vi "Read.vi"(6 "Append Index":i32, 8 "error in (no error)":errorcluster, 11 "DAT in":refnum<class "Data.DAT.lvclass">) -> (0 "error out":errorcluster, 1 "Notes":string, 2 "Data (Dictionary)":T1[](array[typedef]), 3 "DAT out":refnum<class "Data.DAT.lvclass">, 5 "Path out":path)   [LabVIEW 2020, in "Data.DAT.lvclass"]
uses:
  Data.DAT.lvclass
  Data/Data.lvclass
  <vilib>/Utility/file.llb/Read Delimited Spreadsheet (string).vi
  C:/Users/Maya/Documents/GitHub/LV-to-ITX/src/Data/Data.lvclass
  C:/Users/Maya/Documents/GitHub/LV-to-ITX/src/Data.DAT/Data.DAT.lvclass
  Data/Typedefs/Dictionary--cluster.ctl
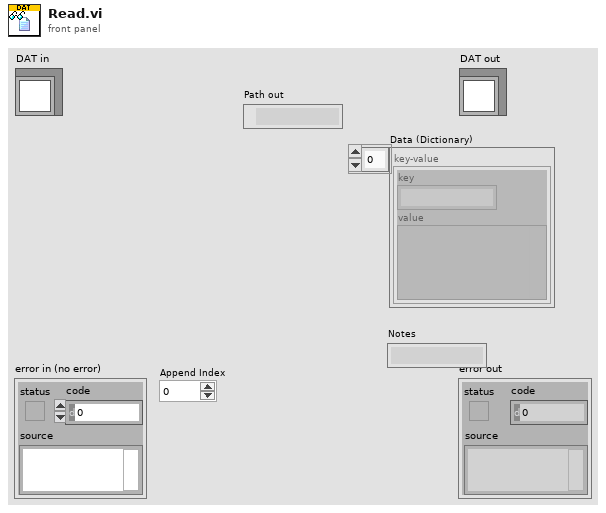
[diagram p1: front panel]
types:
  T1 = typedef "Data.lvclass/Dictionary--cluster.ctl" = cluster{"key":string, "value":variant}
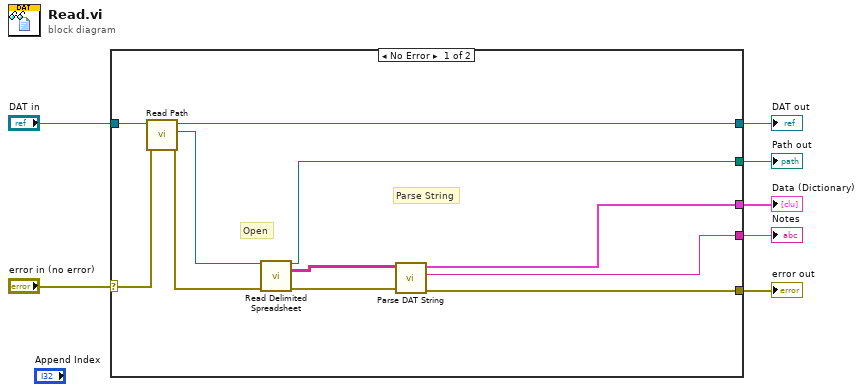
[diagram p0: block diagram]
diagram:
  n1 = case shown="No Error" "error in (no error)" {
    selector: "error in (no error)" -> [w11 w20]
    tunnel: "DAT in" -> [w12 w19]
    tunnel: [w16 w19] -> w6
    tunnel: [w15 w20] -> w5
    tunnel: [w10 _] -> w3
    tunnel: [w9 _] -> w2
    tunnel: [w8 _] -> w1
    frame No Error {
      # "Parse String"
      # "Open"
      n2 = call "Read Path.vi"("error in (no error)"=w11, "Data Save"=w12) -> ("error out"=w17:errorcluster, "Path"=w14:path, "Data Save out"=w16:refnum<class "Data.DAT.lvclass">)  [unwired: 7 in]
      n3 = call-poly <vilib>:"Read Delimited Spreadsheet.vi"("file path (dialog if empty)"=w14, "error in (no error)"=w17) -> ("new file path (Not A Path if cancelled)"=w10:path, "all rows"=w13:string[][], "error out"=w18:errorcluster)  [unwired: 8 in, 3 out]
      n4 = call "Parse DAT String.vi"("error in (no error)"=w18, "spreadsheet string"=w13) -> ("error out"=w15:errorcluster, "Notes"=w8:string, "Data (Dictionary)"=w9:T1[])  [unwired: 7 in]
    }
    frame Error {
    }
  }
  "error out" <- w5
  "DAT out" <- w6
  "Path out" <- w3
  "Data (Dictionary)" <- w2
  "Notes" <- w1
